vi "ResonanceAnalyzer.vi"() -> ()   [LabVIEW 2014]
uses:
  <vilib>/imath/engines/lvmath2/RunTimeEngine/Managers/WorkSpace/UID Generator.vi
  <vilib>/imath/engines/lvmath2/RunTimeEngine/RangeToken/NIMS_Range.vi
  <vilib>/imathl/engines/lvmath/Functions/Error Handling/Create Error.vi
  <vilib>/imath/engines/lvmath2/RunTimeEngine/LocalVariableDefStatement/MC_LocalVariableDefStatement_Display.vi
  <vilib>/imath/engines/lvmath2/RunTimeEngine/RunTimeType/NIMS_RunTimeType_From StrictType (excl LVString).vi
  <vilib>/imath/engines/lvmath2/RunTimeEngine/ArithmeticOperatorToken/NIMS_ArithmeticOperator_minus.vi
  <vilib>/imath/engines/lvmath2/RunTimeEngine/BuiltInFunctions/size/NIMS_I32Row=size(GRow).vi
  <vilib>/imath/engines/lvmath2/RunTimeEngine/BuiltInFunctions/randnormal/NIMS_randnormal(I32V).vi
  <vilib>/imath/engines/lvmath2/RunTimeEngine/ErrorHandling/NIMS_Create Error From Enums.vi
  <vilib>/imath/engines/lvmath2/RunTimeEngine/ArithmeticOperatorToken/NIMS_ArithmeticOperator_plus.vi
  <vilib>/imath/engines/lvmath2/RunTimeEngine/NodeEndStatement/NIMS_NodeEndStatement_Get Vector.vi
  <vilib>/imath/engines/lvmath2/RunTimeEngine/Managers/SymbolTable/Clear UID.vi
  <vilib>/imath/engines/lvmath2/RunTimeEngine/Managers/SymbolTable/NIMS_WorkSpace.lvlib
  <vilib>/imath/engines/lvmath/Functions/Error Handling/MergeErrorsWrapper.vi
  <vilib>/imath/engines/lvmath2/RunTimeEngine/NodeEndStatement/NIMS_NodeEndStatement_Output.vi
  <vilib>/imath/engines/lvmath2/RunTimeEngine/ErrorHandling/NIMS_Finalize Error.vi
  <vilib>/gmath/NI_Gmath.lvlib
  <vilib>/gmath/NumericalOptimization/Nonlinear Curve Fit LM.vi
panel:
  in  "initial parameters":dbl[](array[numeric])
  out "best fit parameters":dbl[](array[numeric])
  in  "best fit":dbl
  out "XY Graph":cluster{"all rows":dbl[], "all rows":dbl[]}(graph)={"all rows"=[400.0, 405.0, 410.0, 415.0, 420.0, 425.0, 430.0, 435.0, 440.0, 445.0, 450.0, 455.0, 460.0, 465.0, 470.0, 475.0, 480.0, 485.0, 490.0, 495.0, 500.0, 505.0, 510.0, 515.0, 520.0, 525.0, 530.0, 535.0, 540.0, 545.0, 550.0, 555.0, 560.0, 565.0, 570.0, 575.0, 580.0, 585.0, 590.0, 595.0, 600.0, 605.0, 610.0, 615.0, 620.0, 625.0, 630.0, 635.0, 640.0, 645.0, 650.0, 655.0, 660.0, 665.0, 670.0, 675.0, 680.0, 685.0, 690.0, 695.0, 700.0, 705.0, 710.0, 715.0, 720.0, 725.0, 730.0, 735.0, 740.0, 745.0, 750.0, 755.0, 760.0, 765.0, 770.0, 775.0, 780.0, 785.0, 790.0, 795.0, 800.0], "all rows"=[0.10905835222346522, 0.12548757267645297, 0.11505297644299414, 0.1409656441240317, 0.14222684793880266, 0.1453211079553719, 0.13321904483293623, 0.15314997861241583, 0.15737373775573787, 0.14260212231431543, 0.1797616146058344, 0.1770714539599552, 0.19455095355756938, 0.20484188761683372, 0.21303301593522977, 0.21946683391382926, 0.21905365642477673, 0.22771607049488085, 0.24038509776020286, 0.25484848883177885, 0.26197263926596037, 0.2714011453464934, 0.283471704919934, 0.3236680071048905, 0.332785704083823, 0.36151942491251177, 0.38439800222876797, 0.39116184213367905, 0.41942032306693366, 0.45826162759907607, 0.49243245993614365, 0.5406201780350152, 0.5885019693939663, 0.6367922647438887, 0.6775132095439435, 0.7665363120960343, 0.8297686100407691, 0.8919909012143868, 0.9512377694698578, 0.9747870210782836, 0.994517241365649, 0.9896257704208898, 0.9531525362778683, 0.8907202651999421, 0.8372569296569699, 0.7604721808398842, 0.7225331129049276, 0.6613825578093208, 0.6102912240462107, 0.5707608368815278, 0.5275282733457685, 0.5157501768871737, 0.4919226019728976, 0.43940339779827975, 0.42673929945694156, 0.38753545712673154, 0.3718407550769163, 0.3675568580995603, 0.34464129933577725, 0.3135333087108802, 0.31435050689156535, 0.288345205625331, 0.2698472433607259, 0.2806399094554873, 0.25219886034469485, 0.2615452362238207, 0.24163435078254272, 0.22869868799002857, 0.22947866470101602, 0.22396957723228747, 0.2094896033951032, 0.20812004298731274, 0.21896627617005554, 0.21765369562732012, 0.1880994086875111, 0.1871863596305589, 0.18289063921809082, 0.1978424481692749, 0.14868654077900095, 0.18060611753242814, 0.17147511699395768]}
  in  "Tab Control":enum32{"Simulation", "Experiment"}(tab)
  in  "Q":i32=10
  in  "Center Frequency":i32=600
  in  "Start Frequency":i32=400
  in  "End Frequency":i32=800
  in  "df":i32=5
  in  "Noise Level":dbl=0.01
  in  "Path":path
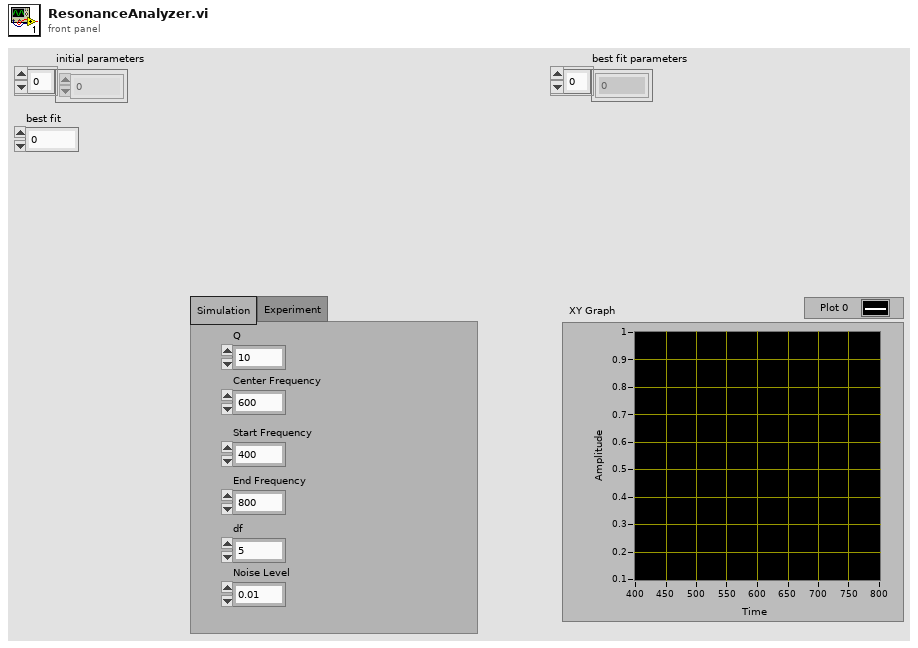
[diagram p1: front panel]
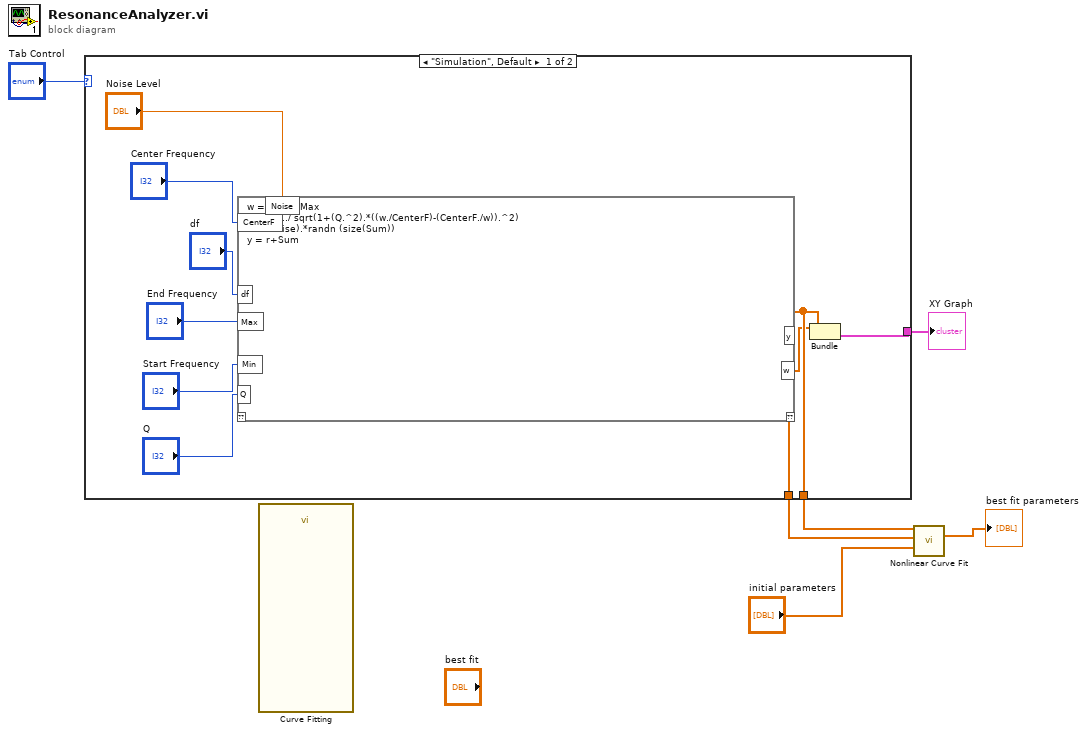
[diagram p0: block diagram]
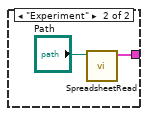
[diagram p2: hidden frame]
diagram:
  n1 = case shown="\"Simulation\", Default" "Tab Control" {
    tunnel: [w9 w176] -> w5
    tunnel: [w8 _] -> w4
    tunnel: [w7 _] -> w3
    frame "Simulation", Default {
      n2 = mathscript code="w = Min:df:Max\nSum =1./ sqrt(1+(Q.^2).*((w./CenterF)-(CenterF./w)).^2)\nr = (Noise).*randn (size(Sum))\ny = r+Sum"("Min"="Start Frequency", "Max"="End Frequency", "df"="df", "Q"="Q", "CenterF"="Center Frequency", "Noise"="Noise Level") -> ("y"=w8:dbl[], "w"=w7:dbl[])  [unwired: 1 in, 1 out]
      n3 = Bundle("w"=w7, "y"=w8) -> (w9:cluster{"w":dbl[], "y":dbl[]})  [unwired: 1 in]
    }
    frame "Experiment" {
      n4 = call "SpreadsheetRead.vi"("Path"="Path") -> ("XY Graph"=w176:cluster{"all rows":dbl[], "all rows":dbl[]})  [unwired: 10 in]
    }
  }
  "XY Graph" <- w5
  n5 = call "Curve Fitting"() -> ()  [unwired: 7 in, 5 out]
  n6 = call-poly <vilib>:"Nonlinear Curve Fit.vi"("Y"=w4, "X"=w3, "initial parameters"="initial parameters") -> ("best fit parameters"=→"best fit parameters":dbl[])  [unwired: 7 in, 5 out]
